vi "JSON Match.vi"(8 "error in (no error)":errorcluster, 10 "JSON Token":T1=enum."comma", 11 "Alpaca CLI Parser in":refnum<class "JSON Parser.lvclass">) -> (0 "error out":errorcluster, 3 "Alpaca CLI Parser out":refnum<class "JSON Parser.lvclass">)   [LabVIEW 2013, in "JKI JSON Serialization.lvlib" / "JSON Parser.lvclass"]
uses:
  JSON Parser.lvclass
  JSON Lexer/JSON Token Type.ctl
  JSON Lexer/JSON Lexer.lvclass
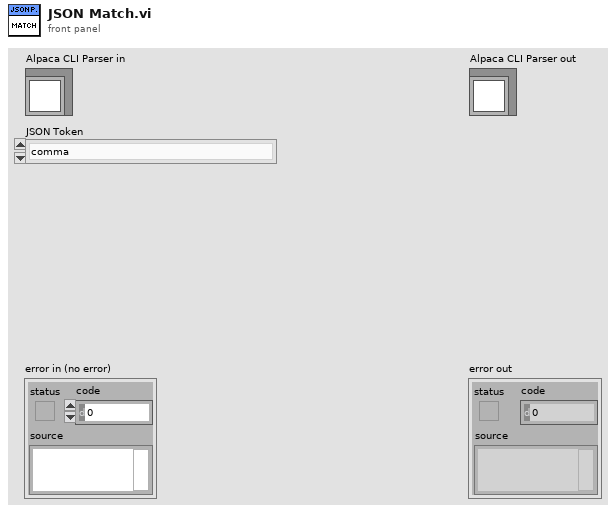
[diagram p1: front panel]
types:
  T1 = typedef "JKI JSON Serialization.lvlib/JSON Lexer.lvclass/JSON Token Type.ctl" = enum32{"unknown", "comma", "end-label", "begin-object", "end-object", "begin-array", "end-array", "quoted-string", "boolean", "exponential-number", "decimal-number", "integer-number", "special-number", "null", "symbol", "whitespace", "EOF"}
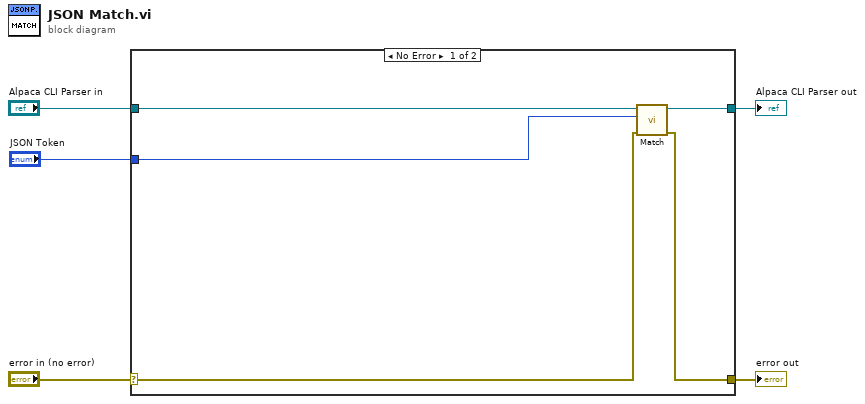
[diagram p0: block diagram]
diagram:
  n1 = case shown="No Error" "error in (no error)" {
    selector: "error in (no error)" -> [w7 w12]
    tunnel: [w9 w12] -> w4
    tunnel: [w10 w11] -> w2
    tunnel: "Alpaca CLI Parser in" -> [w8 w11]
    tunnel: "JSON Token" -> [w6 _]
    frame No Error {
      n2 = call-dynamic "Match.vi"("error in (no error)"=w7, "Token Type"=w6, "Alpaca Parser in"=w8) -> ("error out"=w9:errorcluster, "Alpaca Parser out"=w10:refnum<class "JSON Parser.lvclass">)  [unwired: 7 in]
    }
    frame Error {
    }
  }
  "error out" <- w4
  "Alpaca CLI Parser out" <- w2
